vi "GUI Properties.vi"(4 "GUI":refnum<vi>) -> (7 "GUI Properties":T1)   [LabVIEW 2020, in "VolatusGUI.lvlib" / "GUI Helper.lvclass"]
uses:
  GUI Helper.lvclass
  GUI Properties.ctl
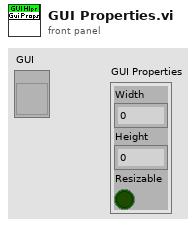
[diagram p1: front panel]
types:
  T1 = typedef "VolatusGUI.lvlib/GUI Helper.lvclass/GUI Properties.ctl" = cluster{"Width":u16, "Height":u16, "Resizable":bool}
  T2 = typedef "LVRectTypeDef.ctl" = cluster{"Left":i16, "Top":i16, "Right":i16, "Bottom":i16}
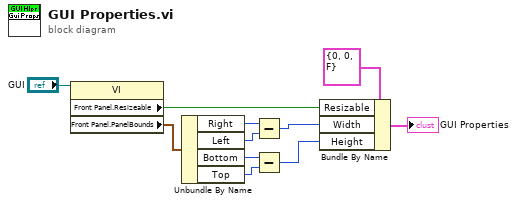
[diagram p0: block diagram]
diagram:
  n1 = property class="VI"(reference="GUI") -> ("Front Panel.Resizeable"=w8:bool, "Front Panel.PanelBounds"=w10:T2)  [unwired: 1 in, 2 out]
  n2 = Unbundle By Name(w10) -> ("Right"=w7:i16, "Left"=w6:i16, "Bottom"=w5:i16, "Top"=w4:i16)
  n3 = Subtract(x=w7, y=w6) -> (x-y=w3:i16)
  n4 = Subtract(x=w5, y=w4) -> (x-y=w2:i16)
  n5 = Bundle By Name(cluster=T1 {"Width"=0, "Height"=0, "Resizable"=FALSE} ("GUI Properties"), "Resizable"=w8, "Width"=w3, "Height"=w2) -> (→"GUI Properties":T1)
